vi "ReadCSVwithQuotes.vi"(8 "error in (no error)":errorcluster, 11 "File Path":path) -> (0 "error out":errorcluster, 2 "Array":string[][](array[string]), 3 "File Path out":path)   [LabVIEW 2025, in "Test Limits.lvlib"]
uses:
  Test Limits.lvlib
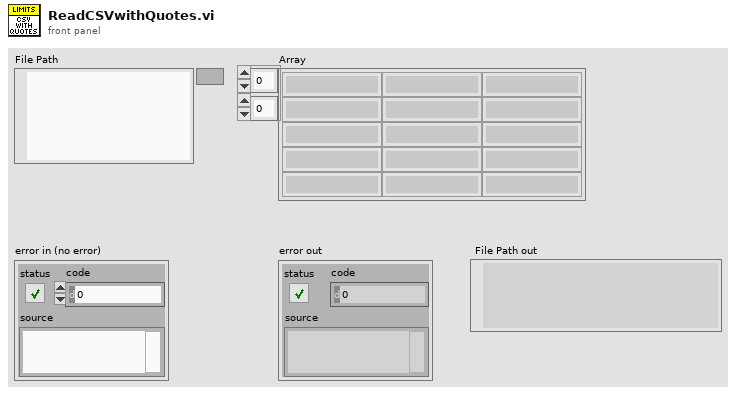
[diagram p1: front panel]
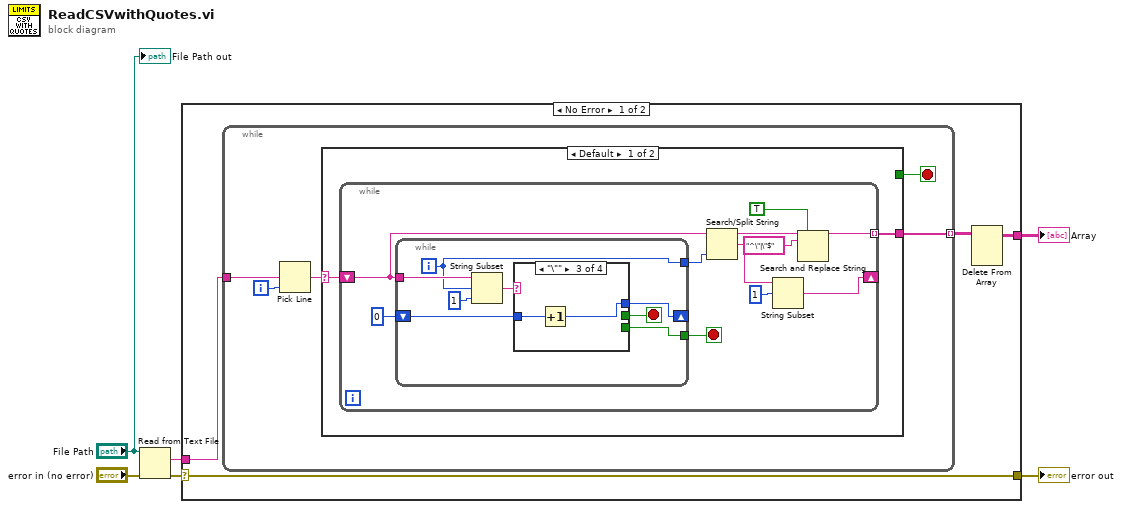
[diagram p0: block diagram]
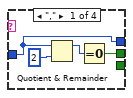
[diagram p2: hidden frame]
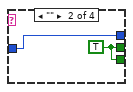
[diagram p3: hidden frame]
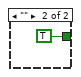
[diagram p5: hidden frame]
diagram:
  n1 = Read from Text File(file (use dialog)="File Path", error in="error in (no error)") -> (text=w5:string, error out=w3:errorcluster)  [unwired: 2 in, 2 out]
  n2 = case shown="No Error" w3 {
    selector: w3 -> [w7 w47]
    tunnel: [w9 _] -> w6
    tunnel: w5 -> [w8 _]
    tunnel: [w7 w47] -> w2
    frame No Error {
      n3 = while {
        tunnel: w8 -> [w14]
        tunnel: [w11] -> w10 mode=indexing
        i -> [w15]
        stop <- w12 stop-if-true
        n4 = Pick Line(multi-line string=w14, line index=w15) -> (output string=w13:string)  [unwired: 1 in]
        n5 = case shown="Default" w13 {
          selector: w13 -> [w17 _]
          tunnel: [_ TRUE] -> w12
          tunnel: [w16 _] -> w11
          frame Default {
            n6 = while {
              tunnel: [w20] -> w16 mode=indexing
              shift-right: [w22] -> _
              shift-left: w17 -> [w27]
              stop <- w26 stop-if-true
              n7 = while {
                tunnel: w27 -> [w31]
                shift-right: [w33] -> _
                shift-left: 0 -> [w34]
                tunnel: [w30] -> w26
                tunnel: [w29] -> w25
                i -> [w29]
                stop <- w32 stop-if-true
                n8 = String Subset(string=w31, offset (0)=w29, length (rest)=1 ("length (rest)")) -> (substring=w35:string)
                n9 = case shown="\"\\\"\"" w35 {
                  tunnel: w34 -> [w40 w41 w44 w45]
                  tunnel: [w40 w41 w43 w45] -> w33
                  tunnel: [w37 w42 _ _] -> w32
                  tunnel: [_ w42 _ _] -> w30
                  frame "," {
                    n10 = Quotient & Remainder(x=w40, y=2) -> (x-y*floor(x/y)=w38:i32)  [unwired: 1 out]
                    n11 = Equal To 0?(x=w38) -> (x = 0?=w37:bool)
                  }
                  frame "" {
                    w42 = TRUE
                  }
                  frame "\"" {
                    n12 = Increment(x=w44) -> (x+1=w43:i32)
                  }
                  frame Default {
                  }
                }
              }
              n13 = Search/Split String(string=w27, offset (0)=w25) -> (substring before match=w21:string, match + rest of string=w24:string)  [unwired: 1 in, 1 out]
              n14 = String Subset(string=w24, offset (0)=1) -> (substring=w22:string)  [unwired: 1 in]
              n15 = Search and Replace String(replace all?=TRUE ("replace all? (F)"), input string=w21, search string="^\"|\"$") -> (result string=w20:string)  [unwired: 5 in, 3 out]
            }
          }
          frame "" {
          }
        }
      }
      n16 = Delete From Array(array=w10) -> (array with subset deleted=w9:string[][])  [unwired: 3 in, 1 out]
    }
    frame Error {
    }
  }
  "Array" <- w6
  "error out" <- w2
  "File Path out" <- "File Path"
